vi "Handle Loop Errors.vi"(8 "error in":errorcluster) -> (0 "error out":errorcluster)   [LabVIEW 2022 SP3]
doc: "Handles Loop Errors\n\nIf \"error in\" contains no error, this VI does nothing.\nIf \"error in\" contains an error, this VI pops that error up as a one button dialogue, and then clears the error."
panel:
  # "Development\ncontrols/indicators useful for development and testing, but which are not outputs of the VI"
  # "Input\nInputs to the VI"
  # "Output\nOutputs of the VI"
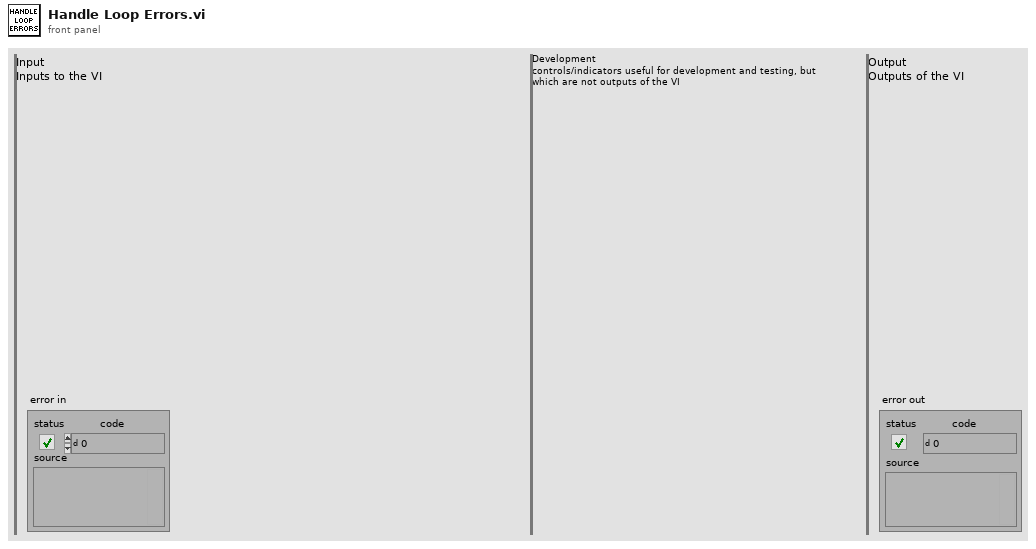
[diagram p1: front panel]
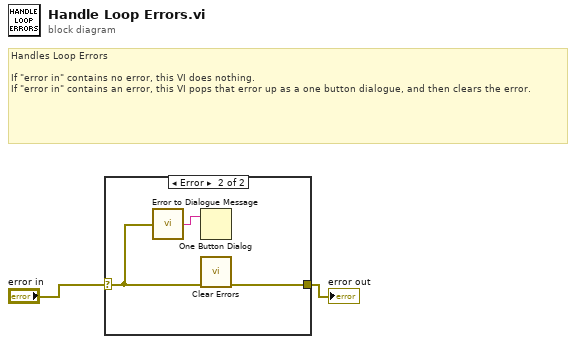
[diagram p0: block diagram]
diagram:
  # "Handles Loop Errors\n\nIf \"error in\" contains no error, this VI does nothing.\nIf \"error in\" contains an error, this VI pops that error up as a one button dialogue, and then clears the error."
  n1 = case shown="Error" "error in" {
    selector: "error in" -> [w3 w6]
    tunnel: [w3 w4] -> w1
    frame No Error {
      # "Do nothing."
    }
    frame Error {
      n2 = call "Error to Dialogue Message.vi"("error in"=w6) -> ("Dialogue Message"=w5:string)
      n3 = One Button Dialog(message=w5) -> ()  [unwired: 1 in, 1 out]
      n4 = call <vilib>:"Clear Errors.vi"("error in (no error)"=w6) -> ("error out"=w4:errorcluster)  [unwired: 5 in, 1 out]
    }
  }
  "error out" <- w1
